vi "Global 1.vi"() -> ()   [LabVIEW 2017]
panel:
  in  "Time":i64
  in  "Stop flage":bool
  in  "ohm refe flage":bool
  in  "measure type":dbl
  in  "Append flage":bool
  in  "APP INDEX":i32=5000000 format="%#.6g"
  in  "Timeout (10000 ms)":i32=5000000 format="%#.6g"
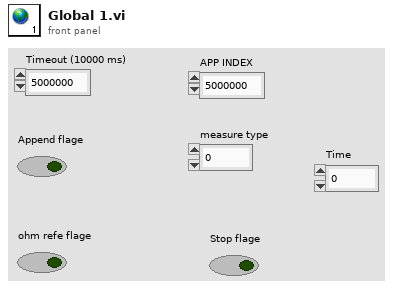
[diagram p1: front panel]
diagram:
